vi "XYZ Stage-Response parser for coordinates.vi"(11 "Filtered response string (no CR)":string="111\t333\t444") -> (1 "Z":sgl, 2 "Y":sgl, 3 "X":sgl)   [LabVIEW 2013]
panel:
  out "before substring 3":string
  out "before substring 2":string
  out "match substring":string
  out "before substring 1":string
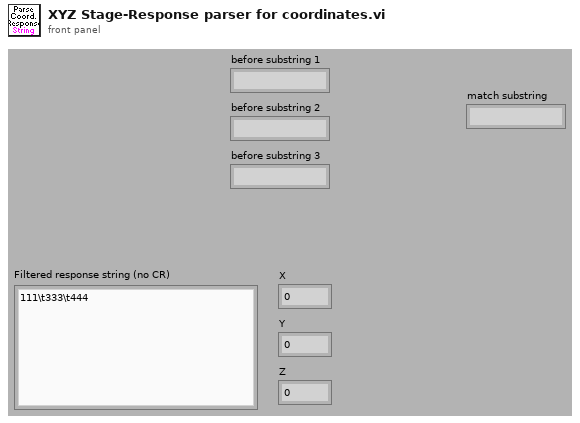
[diagram p1: front panel]
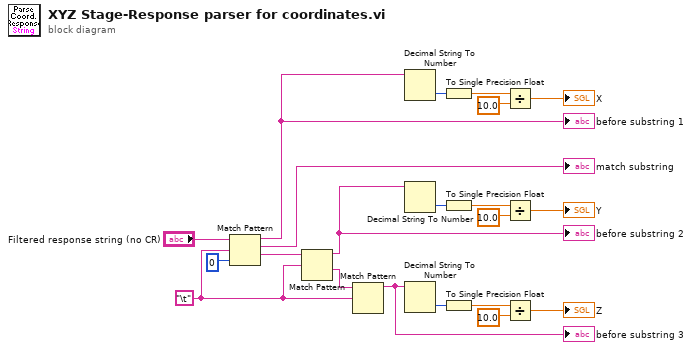
[diagram p0: block diagram]
diagram:
  w17 = "\t"
  n1 = Match Pattern(string="Filtered response string (no CR)", regular expression=w17, offset (0)=0) -> (before substring=w15:string, match substring=→"match substring":string, after substring=w18:string)  [unwired: 1 out]
  "before substring 1" <- w15
  n2 = Match Pattern(string=w18, regular expression=w17) -> (before substring=w14:string, after substring=w16:string)  [unwired: 1 in, 2 out]
  "before substring 2" <- w14
  n3 = Match Pattern(string=w16, regular expression=w17) -> (before substring=w13:string)  [unwired: 1 in, 3 out]
  "before substring 3" <- w13
  n4 = Decimal String To Number(string=w15) -> (number=w12:i32)  [unwired: 2 in, 1 out]
  n5 = Decimal String To Number(string=w14) -> (number=w9:i32)  [unwired: 2 in, 1 out]
  n6 = Decimal String To Number(string=w13) -> (number=w7:i32)  [unwired: 2 in, 1 out]
  n7 = To Single Precision Float(number=w12) -> (single precision float=w1:sgl)
  n8 = To Single Precision Float(number=w9) -> (single precision float=w2:sgl)
  n9 = To Single Precision Float(number=w7) -> (single precision float=w3:sgl)
  n10 = Divide(x=w1, y=sgl 10.0) -> (x/y=→"X":sgl)
  n11 = Divide(x=w2, y=sgl 10.0) -> (x/y=→"Y":sgl)
  n12 = Divide(x=w3, y=sgl 10.0) -> (x/y=→"Z":sgl)
